vi "GNSS Read.vi"(8 "Measurement In":refnum<data-value>, 10 "GNSS Handle":T1, 11 "Error In":errorcluster) -> (0 "Measurement Out":refnum<data-value>, 1 "GNSS Data":T2, 3 "Error Out":errorcluster)   [LabVIEW 2021]
uses:
  GNSS Data.ctl
  GNSS Handle.ctl
  State Estimator/Measurements.ctl
  IMU/IMU Data.ctl
  Steering Motor Encoder/Steering Motor Encoder Data.ctl
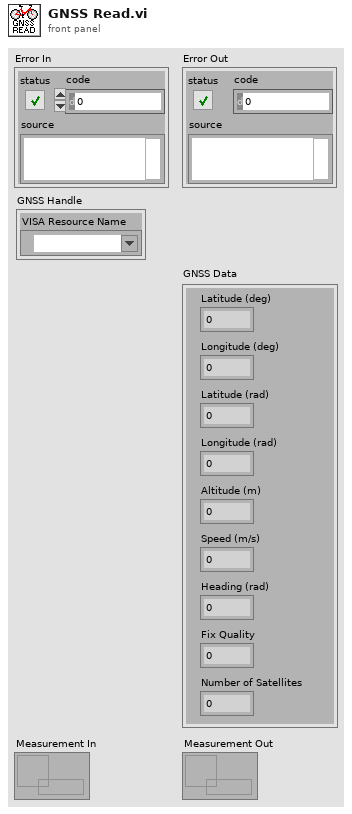
[diagram p1: front panel]
types:
  T1 = typedef "GNSS Handle.ctl" = cluster{"VISA Resource Name":refnum<visa-resource-name>}
  T2 = typedef "GNSS Data.ctl" = cluster{"Latitude (rad)":dbl, "Longitude (rad)":dbl, "Altitude (m)":dbl, "Speed (m/s)":dbl, "Heading (rad)":dbl, "Fix Quality":i32, "Number of Satellites":i32, "Latitude (deg)":dbl, "Longitude (deg)":dbl}
  T3 = typedef "Measurements.ctl" = cluster{"IMU Data":T4, "Steering Motor Encoder Data":T5, "GNSS Data":T2}
  T4 = typedef "IMU Data.ctl" = cluster{"Gyroscope":cluster{"X (rad/s)":dbl, "Y (rad/s)":dbl, "Z (rad/s)":dbl}, "Accelerometer":cluster{"X (m/s^2)":dbl, "Y (m/s^2)":dbl, "Z (m/s^2)":dbl}}
  T5 = typedef "Steering Motor Encoder Data.ctl" = cluster{"Encoder Position (counts)":i32, "Steering Angle (rad)":dbl}
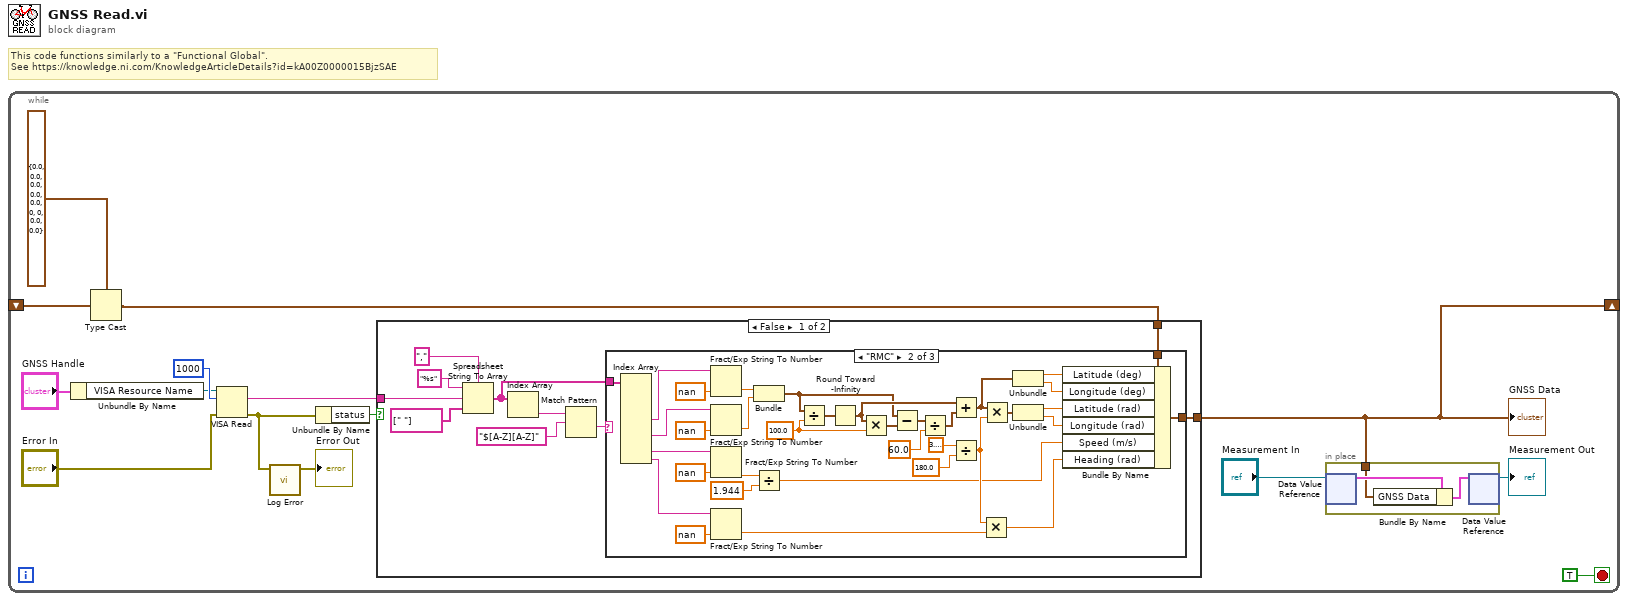
[diagram p0: block diagram]
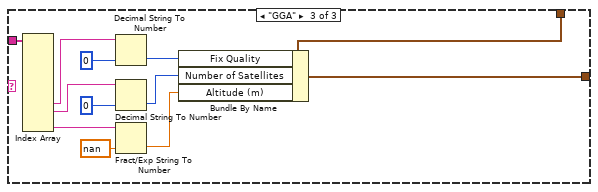
[diagram p3: hidden frame]
diagram:
  # "This code functions similarly to a \"Functional Global\".\nSee https://knowledge.ni.com/KnowledgeArticleDetails?id=kA00Z0000015BjzSAE"
  n1 = while {
    shift-right: [w4] -> _
    shift-left: _ -> [w3]
    stop <- TRUE stop-if-true
    n2 = Unbundle By Name("GNSS Handle") -> ("VISA Resource Name"=w11:refnum<visa-resource-name>)
    n3 = Type Cast(type=T2 {"Latitude (rad)"=0.0, "Longitude (rad)"=0.0, "Altitude (m)"=0.0, "Speed (m/s)"=0.0, "Heading (rad)"=0.0, "Fix Quality"=0, "Number of Satellites"=0, "Latitude (deg)"=0.0, "Longitude (deg)"=0.0} ("GNSS Data 2"), x=w3) -> (*(type *) &x=w2:T2)
    n4 = VISA Read(VISA resource name=w11, byte count=u32 1000, error in (no error)="Error In") -> (read buffer=w14:string, error out=w6:errorcluster)  [unwired: 2 out]
    n5 = call "Log Error.vi"("Error In"=w6) -> ("Error Out"=→"Error Out":errorcluster)  [unwired: 10 in]
    n6 = Unbundle By Name(w6) -> ("status"=w15:bool)
    n7 = case shown="False" w15 {
      tunnel: w14 -> [w28 _]
      tunnel: w2 -> [w20 w77]
      tunnel: [w19 w77] -> w4
      frame False {
        n8 = Spreadsheet String To Array(delimiter (Tab)=",", format string="%s", spreadsheet string=w28, array type (2D Dbl)=string[] [" "]) -> (array=w21:string[])
        n9 = Index Array(array=w21) -> (element=w24:string)  [unwired: 1 in]
        n10 = Match Pattern(string=w24, regular expression="$[A-Z][A-Z]") -> (after substring=w22:string)  [unwired: 1 in, 3 out]
        n11 = case shown="\"RMC\"" w22 {
          tunnel: w21 -> [_ w64 w76]
          tunnel: w20 -> [w29 w35 w66]
          tunnel: [w29 w34 w65] -> w19
          frame Default {
          }
          frame "RMC" {
            w57 = 100.0 ("y")
            n12 = Index Array(array=w64) -> (element #4=w39:string, element #6=w61:string, element #8=w47:string, element #9=w42:string)  [unwired: 9 in, 5 out]
            n13 = Fract/Exp String To Number(string=w39, default (0 dbl)=nan ("default (0 DBL)")) -> (number=w59:dbl)  [unwired: 2 in, 1 out]
            n14 = Fract/Exp String To Number(string=w61, default (0 dbl)=nan ("default (0 DBL)")) -> (number=w60:dbl)  [unwired: 2 in, 1 out]
            n15 = Fract/Exp String To Number(string=w47, default (0 dbl)=nan ("default (0 DBL)")) -> (number=w46:dbl)  [unwired: 2 in, 1 out]
            n16 = Fract/Exp String To Number(string=w42, default (0 dbl)=nan ("default (0 DBL)")) -> (number=w41:dbl)  [unwired: 2 in, 1 out]
            n17 = Bundle(w59, w60) -> (w51:cluster{dbl, dbl})  [unwired: 1 in]
            n18 = Divide(x=w46, y=1.944) -> (x/y=w36:dbl)
            n19 = Divide(x=w51, y=w57) -> (x/y=w58:cluster{dbl, dbl})
            n20 = Round Toward -Infinity(1:w58) -> (0:w53:cluster{dbl, dbl})
            n21 = Multiply(x=w53, y=w57) -> (x*y=w56:cluster{dbl, dbl})
            n22 = Subtract(x=w51, y=w56) -> (x-y=w54:cluster{dbl, dbl})
            n23 = Divide(x=w54, y=60.0) -> (x/y=w52:cluster{dbl, dbl})
            n24 = Add(x=w53, y=w52) -> (x+y=w30:cluster{dbl, dbl})
            n25 = Divide(x=3.141592653589793, y=180.0) -> (x/y=w40:dbl)
            n26 = Multiply(x=w40, y=w41) -> (x*y=w37:dbl)
            n27 = Multiply(x=w30, y=w40) -> (x*y=w48:cluster{dbl, dbl})
            n28 = Unbundle(w30) -> (w32:dbl, w31:dbl)
            n29 = Unbundle(w48) -> (w33:dbl, w38:dbl)
            n30 = Bundle By Name(cluster=w35, "Latitude (deg)"=w32, "Longitude (deg)"=w31, "Latitude (rad)"=w33, "Longitude (rad)"=w38, "Speed (m/s)"=w36, "Heading (rad)"=w37) -> (w34:T2)
          }
          frame "GGA" {
            n31 = Index Array(array=w76) -> (element #7=w75:string, element #8=w74:string, element #10=w73:string)  [unwired: 10 in, 7 out]
            n32 = Decimal String To Number(string=w75, default (0L)=0 ("default (0 I32)")) -> (number=w69:i32)  [unwired: 1 in, 1 out]
            n33 = Decimal String To Number(string=w74, default (0L)=0 ("default (0 I32)")) -> (number=w68:i32)  [unwired: 1 in, 1 out]
            n34 = Fract/Exp String To Number(string=w73, default (0 dbl)=nan ("default (0 DBL)")) -> (number=w67:dbl)  [unwired: 2 in, 1 out]
            n35 = Bundle By Name(cluster=w66, "Fix Quality"=w69, "Number of Satellites"=w68, "Altitude (m)"=w67) -> (w65:T2)
          }
        }
      }
      frame True {
      }
    }
    "GNSS Data" <- w4
    n36 = in-place {
      in-place-border: w4 -> [w16]
      n37 = in-place-dvr #1("Measurement In") -> (w18:T3)  [unwired: 1 out]
      n38 = Bundle By Name(cluster=w18, "GNSS Data"=w16) -> (w17:T3)
      n39 = in-place-dvr #1(w17) -> (→"Measurement Out":refnum<data-value>)  [unwired: 1 out]
    }
  }
